vi "Alarmas_indicadores-LED.vi"() -> ()   [LabVIEW 2018]
panel:
  out "G6_TRANS":bool
  out "G6_SWELL":bool
  out "G6_SAG":bool
  out "G5_TRANS":bool
  out "G5_SWELL":bool
  out "G5_SAG":bool
  out "G4_TRANS":bool
  out "G4_SWELL":bool
  out "G4_SAG":bool
  out "G3_TRANS":bool
  out "G3_SWELL":bool
  out "G3_SAG":bool
  out "G2_TRANS":bool
  out "G2_SWELL":bool
  out "G2_SAG":bool
  out "G1_TRANS":bool
  out "G1_SWELL":bool
  out "G1_SAG":bool
  out "G6_TOL_FREC":bool
  out "G6_TOL_V3_V1":bool
  out "G6_TOL_V2_V3":bool
  out "G6_TOL_V1_V2":bool
  out "G5_TOL_FREC":bool
  out "G5_TOL_V3_V1":bool
  out "G5_TOL_V2_V3":bool
  out "G5_TOL_V1_V2":bool
  out "G4_TOL_FREC":bool
  out "G4_TOL_V3_V1":bool
  out "G4_TOL_V2_V3":bool
  out "G4_TOL_V1_V2":bool
  out "G3_TOL_FREC":bool
  out "G3_TOL_V3_V1":bool
  out "G3_TOL_V2_V3":bool
  out "G3_TOL_V1_V2":bool
  out "G2_TOL_FREC":bool
  out "G2_TOL_V3_V1":bool
  out "G2_TOL_V2_V3":bool
  out "G2_TOL_V1_V2":bool
  out "G1_TOL_FREC":bool
  out "G1_TOL_V3_V1":bool
  out "G1_TOL_V2_V3":bool
  out "G1_TOL_V1_V2":bool
  out "G6_MOD_FREC":bool
  out "G6_MOD_V3_V1":bool
  out "G6_MOD_V2_V3":bool
  out "G6_MOD_V1_V2":bool
  out "G5_MOD_FREC":bool
  out "G5_MOD_V3_V1":bool
  out "G5_MOD_V2_V3":bool
  out "G5_MOD_V1_V2":bool
  out "G4_MOD_FREC":bool
  out "G4_MOD_V3_V1":bool
  out "G4_MOD_V2_V3":bool
  out "G4_MOD_V1_V2":bool
  out "G3_MOD_FREC":bool
  out "G3_MOD_V3_V1":bool
  out "G3_MOD_V2_V3":bool
  out "G3_MOD_V1_V2":bool
  out "G2_MOD_FREC":bool
  out "G2_MOD_V3_V1":bool
  out "G2_MOD_V2_V3":bool
  out "G2_MOD_V1_V2":bool
  out "G1_MOD_FREC":bool
  out "G1_MOD_V3_V1":bool
  out "G1_MOD_V2_V3":bool
  out "G1_MOD_V1_V2":bool
  # "IEEE45"
  # "MODULACION"
  # "TOLERANCIA"
  # "EN 50160"
  # "SAG"
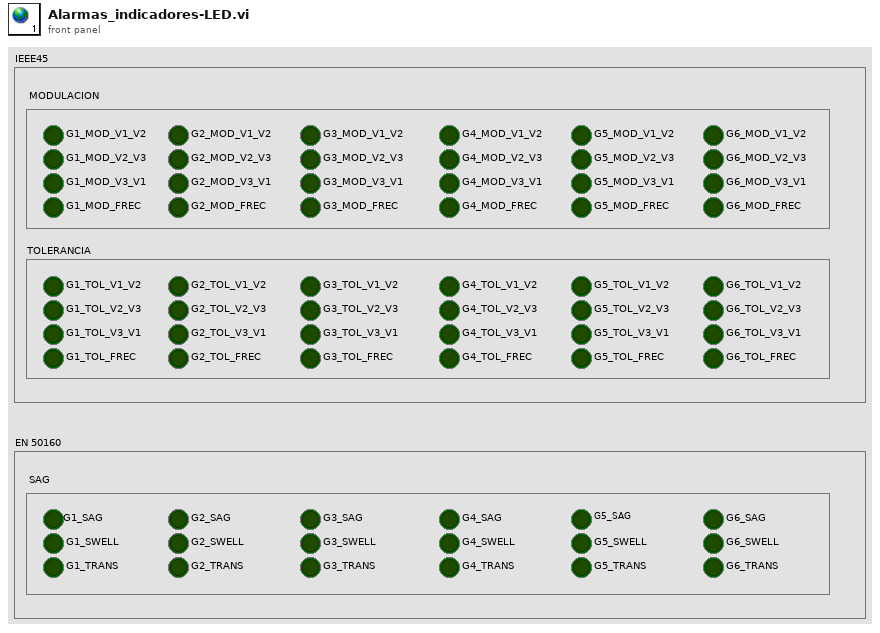
[diagram p1: front panel]
diagram:
